vi "Initialize Driver.vi"(8 "error in (no error)":errorcluster, 11 "Section Ref in":T21 format="%.0x") -> (0 "error out":errorcluster, 3 "Vars":T1 {"OutgoingRegisters.Refs"."Data Type" format="%.0x"; "IncomingDMA.Refs"."Refs"."Data Type" format="%.0x"; "IncomingDMA.Refs"."DMA Settings"."DMA Host Buffer" items=["1 Second"=1, "2 Seconds"=2, "5 Seconds"=5, "10 Seconds"=10]; "IncomingDMA.Refs"."DMA Settings"."dt" format="%#_p"; "IncomingDMA.Refs"."DMA Settings"."Update Rate" items=["1 Hz"=1, "2 Hz"=2, "5 Hz"=5, "10 Hz"=10]; "IncomingRegisters.Refs"."Data Type" format="%.0x"; "OutgoingDMA.Refs"."Refs"."Data Type" format="%.0x"; "Compiled"."IncomingRegisters.Settings"."Register"."Data Type" format="%.0x"; "Compiled"."IncomingRegisters.Refs"."Refs"."Data Reference" format="%.0x"; "Compiled"."OutgoingRegisters.Settings"."Register"."Data Type" format="%.0x"; "Compiled"."OutgoingRegisters.Refs"."Refs"."Data Reference" format="%.0x"; "Compiled"."IncomingDMA.Settings"."Data Type" format="%.0x"; "Compiled"."IncomingDMA.Settings"."DMA.Settings"."DMA Host Buffer" items=["1 Second"=1, "2 Seconds"=2, "5 Seconds"=5, "10 Seconds"=10]; "Compiled"."IncomingDMA.Settings"."DMA.Settings"."dt" format="%#_p"; "Compiled"."IncomingDMA.Settings"."DMA.Settings"."Update Rate" items=["1 Hz"=1, "2 Hz"=2, "5 Hz"=5, "10 Hz"=10]; "Compiled"."OutgoingDMA.Settings"."Data Type" format="%.0x"; "Compiled"."OutgoingDMA.Settings"."DMA.Settings"."DMA Host Buffer" items=["1 Second"=1, "2 Seconds"=2, "5 Seconds"=5, "10 Seconds"=10]; "Compiled"."OutgoingDMA.Settings"."DMA.Settings"."dt" format="%#_p"; "Compiled"."OutgoingDMA.Settings"."DMA.Settings"."Update Rate" items=["1 Hz"=1, "2 Hz"=2, "5 Hz"=5, "10 Hz"=10]})   [LabVIEW 2018, in "FPGA Addon Engine.lvlib"]
uses:
  FPGA Addon Engine.lvlib
  Addon Shared/SubVIs/Constants.vi
  Addon Shared/FPGA Addon Shared.lvlib
  Addon Shared/Types/FG Action.ctl
  <vilib>/NI Veristand/Custom Device API/Data Reference.ctl
  <vilib>/NI Veristand/Custom Device API/Custom Device API.lvlib
  <vilib>/NI Veristand/Custom Device API/Block Data Reference.ctl
  Types/State Variables.ctl
  Addon Shared/Types/Delacing Scheme.ctl
  Addon Shared/Types/DMA Settings.ctl
  <vilib>/NI Veristand/Custom Device Waveform API/Multiple Waveforms Write (DBL)/Multiple Waveforms Write (DBL).lvclass
  Types/Register Settings.ctl
  Addon Shared/Types/Scalar Type.ctl
  <vilib>/NI Veristand/Custom Device API/Waveform Data Reference.ctl
  Types/DMA Input References.ctl
  <vilib>/NI Veristand/Custom Device Waveform API/Single Waveform Read (DBL)/Single Waveform Read (DBL).lvclass
  Types/DMA Output References.ctl
  Addon Shared/Types/FPGA Settings.ctl
  Addon Shared/Types/Compiled.DMASettings.ctl
  Addon Shared/Types/Register Information.ctl
  Addon Shared/Types/Compiled.RegisterSettings.ctl
  Addon Shared/Types/Compiled.Settings.ctl
  Addon Shared/Types/DMA Acquisition Mode.ctl
  <vilib>/NI Veristand/Custom Device API/Custom Device Target Type.ctl
  Addon Shared/Types/FPGA Addon Data Type.ctl
  Types/DMA Input Refs.ctl
  Types/DMA Output Refs.ctl
  <vilib>/NI Veristand/Custom Device API/Get Item Property (Dependent File).vi
  <vilib>/NI Veristand/Custom Device API/Get Item Property (Variant).vi
  <vilib>/NI Veristand/Custom Device API/Custom Device Item Ref.ctl
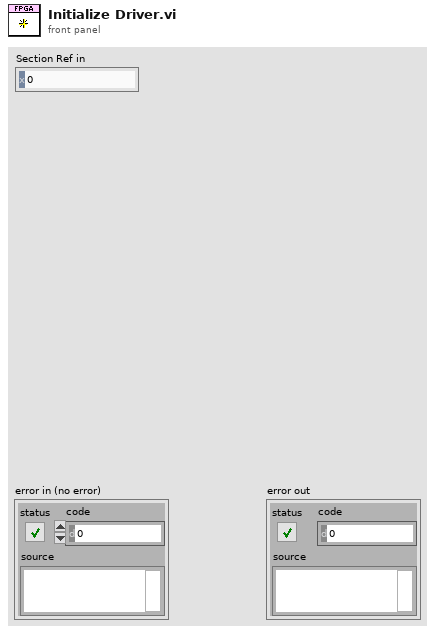
[diagram p1: front panel]
types:
  T1 = typedef "FPGA Addon Engine.lvlib/State Variables.ctl" = cluster{"FPGA Ref":refnum<k20>, "IncomingRegisters.Refs":T2[], "IncomingDMA.Refs":T5[], "OutgoingRegisters.Refs":T2[], "OutgoingDMA.Refs":T10[], "Compiled":T12}
  T2 = typedef "FPGA Addon Engine.lvlib/Register Settings.ctl" = cluster{"Data Type":T3, "U64":refnum<k20>, "U32":refnum<k20>, "U16":refnum<k20>, "U8":refnum<k20>, "I64":refnum<k20>, "I32":refnum<k20>, "I16":refnum<k20>, "I8":refnum<k20>, "SGL":refnum<k20>, "Bool":refnum<k20>, "Scalar Type":T4, "Index":i32, "Length":i32, "Analog PWM In":refnum<k20>, "Digital PWM In":refnum<k20>, "Digital PWM Out":refnum<k20>, "Analog PWM In Settings":refnum<k20>, "Digital PWM In Settings":refnum<k20>, "Sine Out":refnum<k20>, "FXP+/-24.5":refnum<k20>, "FXP+/-16.5":refnum<k20>, "FXP+/-32.8":refnum<k20>, "FXP+/-64.32":refnum<k20>, "FXP+/-16.7":refnum<k20>, "FXP+/-20.5":refnum<k20>, "FXP+/-27.5":refnum<k20>, "FXP+/-32.16":refnum<k20>, "FXP+16.3":refnum<k20>, "FXP+18.3":refnum<k20>, "Digital Static In":refnum<k20>, "Digital Static Out":refnum<k20>, "Digital Static In Settings":refnum<k20>, "Digital WSS Out":refnum<k20>, "Quad Encoder Settings":refnum<k20>, "Quad Encoder In":refnum<k20>}
  T3 = typedef "FPGA Addon Shared.lvlib/FPGA Addon Data Type.ctl" = enum8{"<Null>", "I8", "I16", "I32", "I64", "U8", "U16", "U32", "U64", "SGL", "Boolean", "Analog PWM In Settings", "Analog PWM In", "Digital PWM In Settings", "Digital PWM In", "Digital PWM Out", "Sine Out", "FXP", "FXP+/-24.5", "FXP+/-16.5", "FXP+/-32.8", "FXP+/-64.32", "FXP+/-16.7", "FXP+/-20.5", "FXP+/-27.5", "FXP+/-32.16", "FXP+16.3", "FXP+18.3", "Digital Static In", "Digital Static Out", "Digital Static In Settings", "Digital WSS Out", "Quad Encoder Settings", "Quad Encoder In", "Group"}
  T4 = typedef "FPGA Addon Shared.lvlib/Scalar Type.ctl" = enum16{"Standard", "Bitpacked"}
  T5 = typedef "FPGA Addon Engine.lvlib/DMA Input References.ctl" = cluster{"Addon Name":string, "Waveform Ref":refnum<class "Multiple Waveforms Write (DBL).lvclass">, "DMA Name":string, "DMA Settings":T6, "Refs":T9}
  T6 = typedef "FPGA Addon Shared.lvlib/DMA Settings.ctl" = cluster{"Number of Channels":u8, "Delacing Scheme":T7, "Update Rate":u32, "dt":dbl, "Mode":T8, "Number of Samples":u32, "DMA Host Buffer":u32}
  T7 = typedef "FPGA Addon Shared.lvlib/Delacing Scheme.ctl" = enum8{"Interleaved", "Bitpacked"}
  T8 = typedef "FPGA Addon Shared.lvlib/DMA Acquisition Mode.ctl" = enum8{"Continuous", "Triggered Finite"}
  T9 = typedef "FPGA Addon Engine.lvlib/DMA Input Refs.ctl" = cluster{"Data Type":T3, "DMA_SGL":refnum<k20>, "DMA_U64":refnum<k20>, "DMA_I64":refnum<k20>, "DMA_FXP+/-32.8":refnum<k20>, "DMA_FXP+/-64.32":refnum<k20>, "DMA_U32":refnum<k20>, "DMA_U16":refnum<k20>, "DMA_U8":refnum<k20>, "DMA_I32":refnum<k20>, "DMA_I16":refnum<k20>, "DMA_I8":refnum<k20>, "DMA_FXP+/-32.16":refnum<k20>}
  T10 = typedef "FPGA Addon Engine.lvlib/DMA Output References.ctl" = cluster{"Addon Name":string, "Waveforms":refnum<class "Single Waveform Read (DBL).lvclass">[], "DMA Name":string, "Refs":T11}
  T11 = typedef "FPGA Addon Engine.lvlib/DMA Output Refs.ctl" = cluster{"Data Type":T3, "DMA_SGL":refnum<k20>, "DMA_U64":refnum<k20>, "DMA_I64":refnum<k20>, "DMA_FXP+/-32.8":refnum<k20>, "DMA_FXP+/-64.32":refnum<k20>, "DMA_U32":refnum<k20>, "DMA_U16":refnum<k20>, "DMA_U8":refnum<k20>, "DMA_I32":refnum<k20>, "DMA_I16":refnum<k20>, "DMA_I8":refnum<k20>, "DMA_FXP+/-32.16":refnum<k20>}
  T12 = typedef "FPGA Addon Shared.lvlib/Compiled.Settings.ctl" = cluster{"Name":string, "IncomingRegisters.Settings":T13[], "IncomingRegisters.Refs":cluster{"Refs":T15[], "Values":dbl[]}, "OutgoingRegisters.Settings":T13[], "OutgoingRegisters.Refs":cluster{"Refs":T15[], "Values":dbl[]}, "Incoming.Size":i32, "Outgoing.Size":i32, "IncomingDMA.Settings":T17[], "OutgoingDMA.Settings":T17[], "FPGA.Settings":T19, "Target.Type":T20}
  T13 = typedef "FPGA Addon Shared.lvlib/Compiled.RegisterSettings.ctl" = cluster{"Scalar Type":T4, "Index":i32, "Length":i32, "Register":T14}
  T14 = typedef "FPGA Addon Shared.lvlib/Register Information.ctl" = cluster{"Name":string, "Data Type":T3, "Default Value":variant}
  T15 = typedef "Custom Device API.lvlib/Block Data Reference.ctl" = cluster{"Data Reference":T16, "Offset":u64, "Length":u64}
  T16 = typedef "Custom Device API.lvlib/Data Reference.ctl" = i32
  T17 = typedef "FPGA Addon Shared.lvlib/Compiled.DMASettings.ctl" = cluster{"Name":string, "Data Type":T3, "DMA.Settings":T6, "DMA.VSRefs":T18[]}
  T18 = typedef "Custom Device API.lvlib/Waveform Data Reference.ctl" = i32
  T19 = typedef "FPGA Addon Shared.lvlib/FPGA Settings.ctl" = cluster{"Bitfile path":path, "RIO Device Address":string, "Group":bool}
  T20 = typedef "Custom Device API.lvlib/Custom Device Target Type.ctl" = enum16{"PharLap", "VxWorks", "Windows", "Linux_32_ARM", "Linux_x64"}
  T21 = typedef "Custom Device API.lvlib/Custom Device Item Ref.ctl" = u64
  T22 = typedef "FPGA Addon Shared.lvlib/FG Action.ctl" = enum8{"GET", "SET"}
  T23 = typedef "Custom Device API.lvlib/Dependent File Optional Info.ctl" = cluster{"Version":string, "RTDestination":path, "ForceDownload":bool, "SupportedTarget":string, "MD5":string}
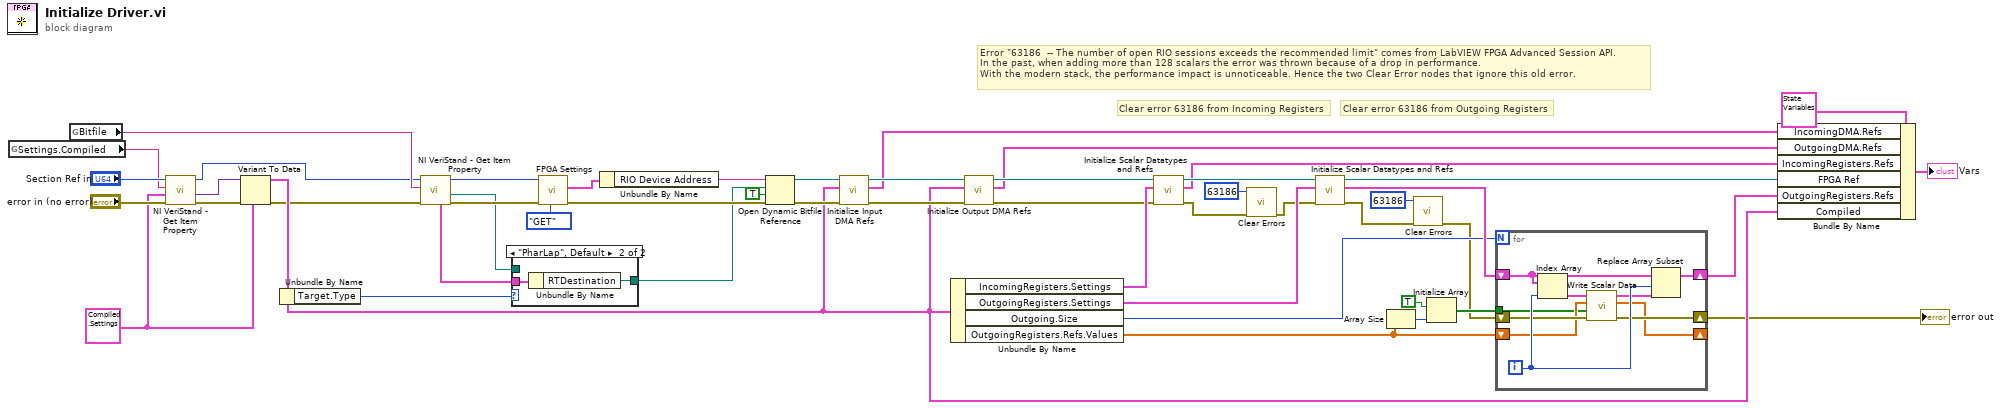
[diagram p0: block diagram]
diagram:
  w19 = T12 {"Name"="", "IncomingRegisters.Settings"=[], "IncomingRegisters.Refs"={"Refs"=[], "Values"=[]}, "OutgoingRegisters.Settings"=[], "OutgoingRegisters.Refs"={"Refs"=[], "Values"=[]}, "Incoming.Size"=0, "Outgoing.Size"=0, "IncomingDMA.Settings"=[], "OutgoingDMA.Settings"=[], "FPGA.Settings"={"Bitfile path"=path "", "RIO Device Address"="", "Group"=FALSE}, "Target.Type"=enum."PharLap"} ("Settings.Compiled")
  # "Clear error 63186 from Outgoing Registers"
  # "Clear error 63186 from Incoming Registers"
  # "Error \"63186  -- The number of open RIO sessions exceeds the recommended limit\" comes from LabVIEW FPGA Advanced Session API.\nIn the past, when adding more than 128 scalars the error was thrown because of a drop in performance.\nWith the modern stack, the performance impact is unnoticeable. Hence the two Clear Error nodes that ignore this old error."
  n1 = global read "Constants.vi" "Settings.Compiled"() -> (w21:string)
  n2 = global read "Constants.vi" "Bitfile"() -> (w43:string)
  n3 = call-poly <vilib>:"NI VeriStand - Get Item Property.vi"("error in (no error)"="error in (no error)", "Default Value"=w19, "Property Name"=w21, "Item Ref in"="Section Ref in") -> ("error out"=w22:errorcluster, "Value"=w20:variant, "Item Ref out"=w15:T21)  [unwired: 4 in, 1 out]
  n4 = Variant To Data(error in=w22, type=w19, Variant=w20) -> (data=w18:T12, error out=w16:errorcluster)
  n5 = Unbundle By Name(w18) -> ("Target.Type"=w17:T20)
  n6 = call-poly <vilib>:"NI VeriStand - Get Item Property.vi"("error in (no error)"=w16, "Property Name"=w43, "Item Ref in"=w15) -> ("error out"=w41:errorcluster, "Path"=w38:path, "Item Ref out"=w42:T21, "OptionalInfo"=w40:T23)  [unwired: 4 in, 1 out]
  n7 = case shown="\"PharLap\", Default" w17 {
    tunnel: w40 -> [_ w53]
    tunnel: [w51 w52] -> w39
    tunnel: w38 -> [w51 _]
    frame "Windows" {
    }
    frame "PharLap", Default {
      n8 = Unbundle By Name(w53) -> ("RTDestination"=w52:path)
    }
  }
  n9 = call "FPGA Settings.vi"("Action"=FG_Action."GET", "error in (no error)"=w41, "Item Ref"=w42) -> ("error out"=w49:errorcluster, "FPGA Settings"=w47:T19)  [unwired: 6 in, 1 out]
  n10 = Unbundle By Name(w47) -> ("RIO Device Address"=w46:string)
  n11 = Open Dynamic Bitfile Reference(0:w46, 1:w39, 2:TRUE ("Run When Loaded"), 3:w49) -> (5:w36:refnum<k20>, 8:w37:errorcluster)  [unwired: 1 in]
  n12 = call "Initialize Input DMA Refs.vi"("error in (no error)"=w37, "Settings.Compiled"=w18, "FPGA Ref"=w36) -> ("error out"=w29:errorcluster, "DMA Settings"=w27:T5[], "FPGA Ref"=w32:refnum<k20>)  [unwired: 6 in]
  n13 = Unbundle By Name(w18) -> ("IncomingRegisters.Settings"=w34:T13[], "OutgoingRegisters.Settings"=w33:T13[], "Outgoing.Size"=w9:i32, "OutgoingRegisters.Refs.Values"=w8:dbl[])
  n14 = call "Initialize Output DMA Refs.vi"("error in (no error)"=w29, "Settings.Compiled"=w18, "FPGA Ref"=w32) -> ("error out"=w30:errorcluster, "DMA"=w26:T10[], "FPGA Ref"=w31:refnum<k20>)  [unwired: 6 in]
  n15 = call "Initialize Scalar Datatypes and Refs.vi"("error in (no error)"=w30, "Registers"=w34, "FPGA Ref"=w31) -> ("error out"=w6:errorcluster, "Registers Ref"=w25:T2[], "FPGA Ref"=w35:refnum<k20>)  [unwired: 6 in]
  n16 = call <vilib>:"Clear Errors.vi"("error in (no error)"=w6, "specific error code to clear (0: all)"=63186) -> ("error out"=w5:errorcluster)  [unwired: 4 in, 1 out]
  n17 = call "Initialize Scalar Datatypes and Refs.vi"("error in (no error)"=w5, "Registers"=w33, "FPGA Ref"=w35) -> ("error out"=w2:errorcluster, "Registers Ref"=w14:T2[], "FPGA Ref"=w28:refnum<k20>)  [unwired: 6 in]
  n18 = Array Size(array=w8) -> (size(s)=w7:i32)
  n19 = call <vilib>:"Clear Errors.vi"("error in (no error)"=w2, "specific error code to clear (0: all)"=63186) -> ("error out"=w1:errorcluster)  [unwired: 4 in, 1 out]
  n20 = Initialize Array(TRUE, w7) -> (w11:bool[])
  n21 = for {
    N: w9 -> [_]
    shift-right: [w55] -> _
    shift-left: w8 -> [w56]
    shift-right: [w63] -> w10
    shift-left: w14 -> [w62]
    shift-right: [w58] -> w13
    shift-left: w1 -> [w59]
    tunnel: w11 -> [w54]
    i -> [w61]
    n22 = Index Array(array=w62, index=w61) -> (element=w57:T2)
    n23 = call "Write Scalar Data.vi"("error in (no error)"=w59, "Changed?"=w54, "Values"=w56, "Cluster"=w57) -> ("error out"=w58:errorcluster, "Values"=w55:dbl[], "Cluster"=w60:T2)  [unwired: 5 in]
    n24 = Replace Array Subset(array=w62, new element=w60, index=w61) -> (w63:T2[])
  }
  "error out" <- w13
  n25 = Bundle By Name(cluster=T1 {"FPGA Ref"=refnum, "IncomingRegisters.Refs"=[], "IncomingDMA.Refs"=[], "OutgoingRegisters.Refs"=[], "OutgoingDMA.Refs"=[], "Compiled"={"Name"="", "IncomingRegisters.Settings"=[], "IncomingRegisters.Refs"={"Refs"=[], "Values"=[]}, "OutgoingRegisters.Settings"=[], "OutgoingRegisters.Refs"={"Refs"=[], "Values"=[]}, "Incoming.Size"=0, "Outgoing.Size"=0, "IncomingDMA.Settings"=[], "OutgoingDMA.Settings"=[], "FPGA.Settings"={"Bitfile path"=path "", "RIO Device Address"="", "Group"=FALSE}, "Target.Type"=enum."PharLap"}}, "IncomingDMA.Refs"=w27, "OutgoingDMA.Refs"=w26, "IncomingRegisters.Refs"=w25, "FPGA Ref"=w28, "OutgoingRegisters.Refs"=w10, "Compiled"=w18) -> (→"Vars":T1)
